vi "Pre SSH Launch Checks.vi"(11 "Connection Info":T1) -> (0 "error out":errorcluster)   [LabVIEW 2017, in "SSH.lvlib"]
doc: "Checks the launch configuration for the new SSH connection and throws an error if its not valid"
uses:
  SSH.lvlib
  Connection Info.ctl
  <vilib>/Utility/error.llb/Error Cluster From Error Code.vi
  <vilib>/ErrorRing/Error Ring.xnode
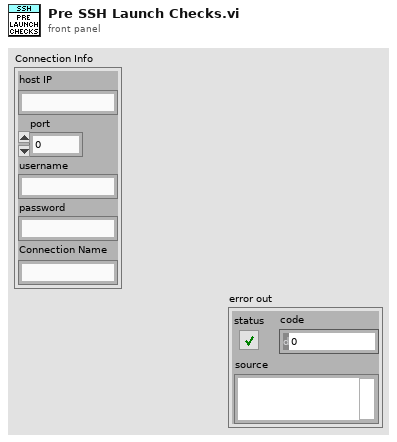
[diagram p1: front panel]
types:
  T1 = typedef "SSH.lvlib/Connection Info.ctl" = cluster{"host IP":string, "port":i32, "username":string, "password":string, "Connection Name":string}
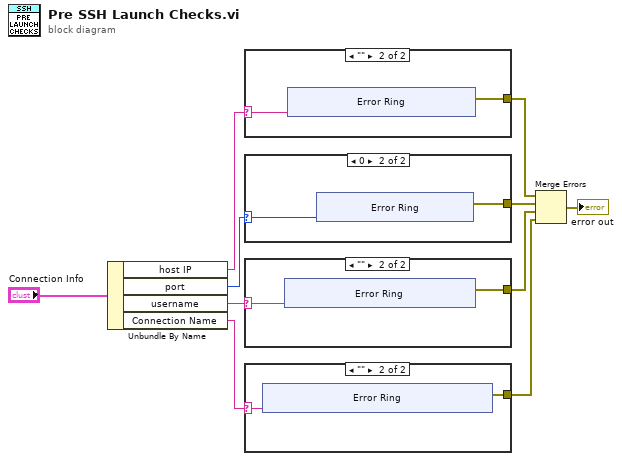
[diagram p0: block diagram]
diagram:
  n1 = Unbundle By Name("Connection Info") -> ("host IP"=w9:string, "port"=w8:i32, "username"=w7:string, "Connection Name"=w6:string)
  n2 = case shown="\"\"" w9 {
    selector: w9 -> [_ w12]
    tunnel: [_ w11] -> w5
    frame Default {
    }
    frame "" {
      n3 = xnode "Error Ring"("parameter 0"=w12) -> ("error out"=w11:errorcluster)
    }
  }
  n4 = case shown="0" w8 {
    selector: w8 -> [_ w21]
    tunnel: [_ w20] -> w4
    frame Default {
    }
    frame 0 {
      n5 = xnode "Error Ring"("parameter 0"=w21) -> ("error out"=w20:errorcluster)
    }
  }
  n6 = case shown="\"\"" w7 {
    selector: w7 -> [_ w30]
    tunnel: [_ w29] -> w3
    frame Default {
    }
    frame "" {
      n7 = xnode "Error Ring"("parameter 0"=w30) -> ("error out"=w29:errorcluster)
    }
  }
  n8 = case shown="\"\"" w6 {
    selector: w6 -> [_ w39]
    tunnel: [_ w38] -> w2
    frame Default {
    }
    frame "" {
      n9 = xnode "Error Ring"("parameter 0"=w39) -> ("error out"=w38:errorcluster)
    }
  }
  n10 = Merge Errors(w5, w4, w3, w2) -> (→"error out":errorcluster)
